vi "UpdateControl.vi"(8 "error in (no error)":errorcluster, 10 "Clust Refnum":refnum<vi>, 11 "Database in":refnum<class "Database.lvclass">) -> (0 "error out":errorcluster, 3 "Database out":refnum<class "Database.lvclass">)   [LabVIEW 2014, in "Database.lvclass"]
uses:
  Database.lvclass
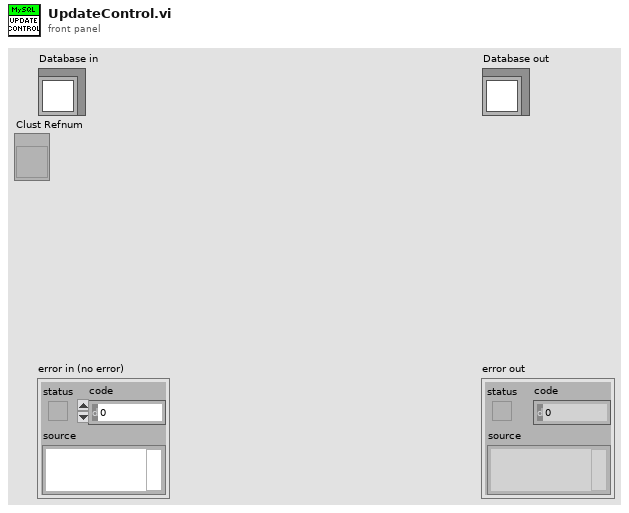
[diagram p1: front panel]
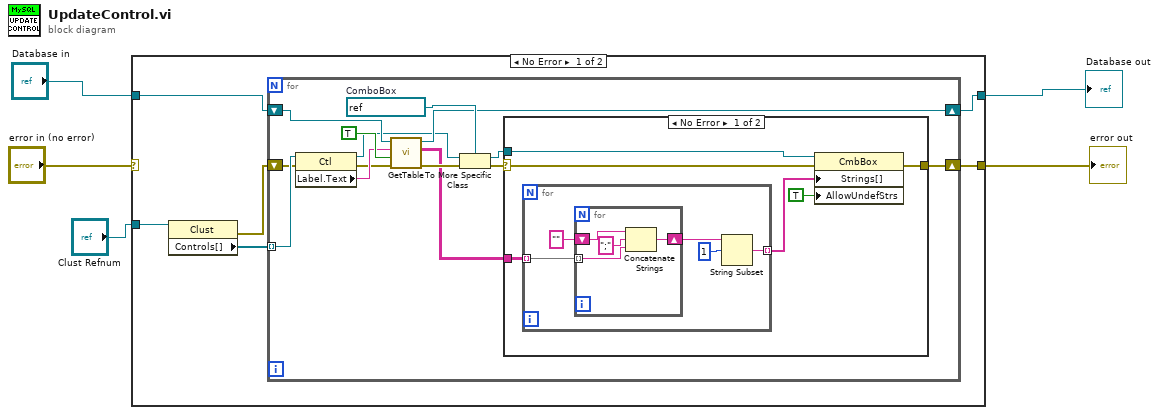
[diagram p0: block diagram]
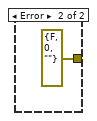
[diagram p2: hidden frame]
diagram:
  n1 = case shown="No Error" "error in (no error)" {
    selector: "error in (no error)" -> [_ w42]
    tunnel: [w7 w43] -> w3
    tunnel: "Database in" -> [w8 w43]
    tunnel: "Clust Refnum" -> [w10 _]
    tunnel: [w6 w42] -> w2
    frame No Error {
      n2 = property class="Clust"(reference=w10) -> (error out=w9:errorcluster, "Controls[]"=w11:refnum<vi>[])  [unwired: 1 in, 1 out]
      n3 = for {
        tunnel: w11 -> [w25] mode=indexing
        shift-right: [w20] -> w7
        shift-left: w8 -> [w21]
        shift-right: [w18] -> w6
        shift-left: w9 -> [w17]
        w24 = refnum<vi> refnum  # ComboBox
        n4 = property class="Ctl"(reference=w25, error in=w17) -> (reference out=w15:refnum<vi>, error out=w16:errorcluster, "Label.Text"=w19:string)
        n5 = call-dynamic "GetTable.vi"("error in (no error)"=w16, "Primary"=TRUE, "table"=w19, "Database in"=w21) -> ("error out"=w14:errorcluster, "data"=w13:string[][], "Database out"=w20:refnum<class "Database.lvclass">)  [unwired: 4 in, 1 out]
        n6 = To More Specific Class(target class=w24, reference=w15, error in=w14) -> (specific class reference=w23:refnum<vi>, error out=w12:errorcluster)
        n7 = case shown="No Error" w12 {
          selector: w12 -> [w26 _]
          tunnel: w23 -> [w31 _]
          tunnel: [w29 errorcluster {"status"=FALSE, "code"=0, "source"=""} ("error out")] -> w18
          tunnel: w13 -> [w28 _]
          frame No Error {
            n8 = for {
              tunnel: w28 -> [w36] mode=indexing
              tunnel: [w32] -> w27 mode=indexing
              n9 = for {
                tunnel: w36 -> [w38] mode=indexing
                shift-right: [w37] -> w34
                shift-left: "" -> [w40]
                n10 = Concatenate Strings(w40, ";" ("string"), w38) -> (w37:string)
              }
              n11 = String Subset(string=w34, offset (0)=1) -> (substring=w32:string)  [unwired: 1 in]
            }
            n12 = property class="CmbBox"(reference=w31, error in=w26, "Strings[]"=w27, "AllowUndefStrs"=TRUE ("Allow Undefined Strings")) -> (error out=w29:errorcluster)  [unwired: 1 out]
          }
          frame Error {
          }
        }
      }
    }
    frame Error {
    }
  }
  "error out" <- w2
  "Database out" <- w3
